vi "Get Configuration in File.vi"(8 "error in":errorcluster, 11 "Configuration File Path":path) -> (0 "error out":errorcluster, 3 "Configuration from File":T1={"Delay Mode"="On", "Trigger Position"=0.0, "Length Unit"="Percentage", "Record Length"=100.0} {"Record Length" format="%#_6g%"; "Trigger Position" format="%#_6ps"})   [LabVIEW 2025, in "Ni-Scope-Multirecords UI.lvlib"]
uses:
  Ni-Scope-Multirecords UI.lvlib
  <vilib>/JDP Science/JSONtext/String Subset.vi
  <vilib>/JDP Science/JSONtext/support/Strip Quotes and Unescape.vi
  <vilib>/JDP Science/JSONtext/support/Unescape JSON string.vi
  <vilib>/JDP Science/JSONtext/Parsing/Parse Full Path or Item Name.vi
  <vilib>/JDP Science/JSONtext/Offset/Find Item Locations by Path.vi
  <vilib>/ErrorRing/Error Ring.xnode
  <vilib>/JDP Science/JSONtext/JSONtext.lvlib
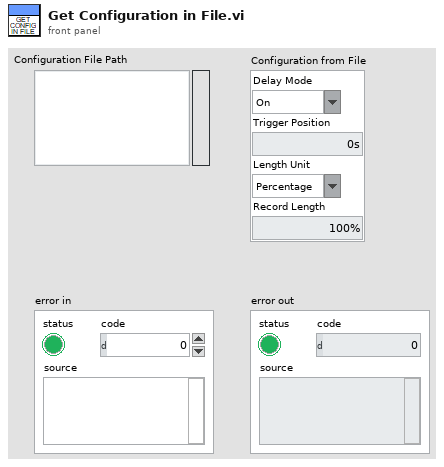
[diagram p1: front panel]
types:
  T1 = cluster{"Delay Mode":string, "Trigger Position":dbl, "Length Unit":string, "Record Length":dbl}
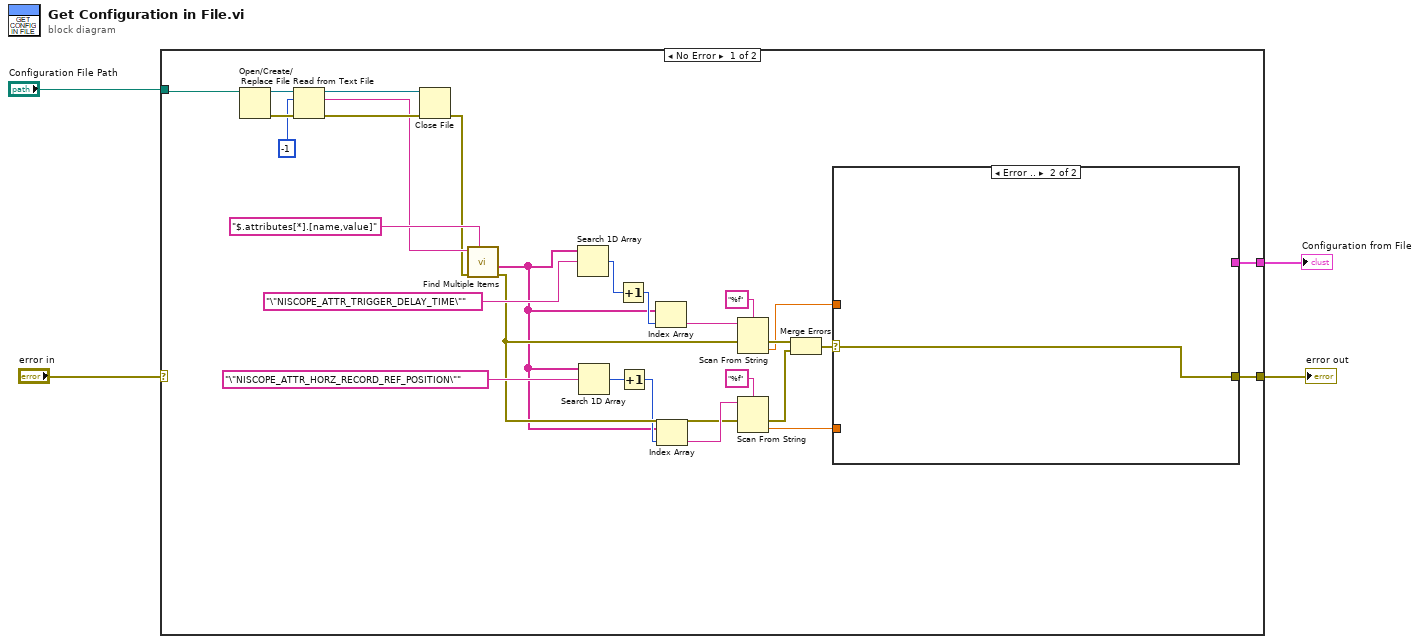
[diagram p0: block diagram]
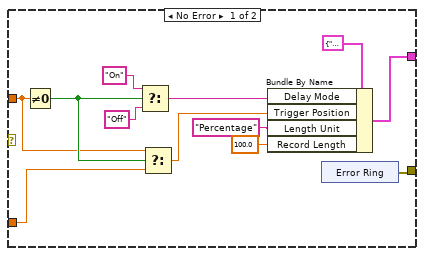
[diagram p2: hidden frame]
diagram:
  n1 = case shown="No Error" "error in" {
    selector: "error in" -> [_ w47]
    tunnel: [w9 w47] -> w3
    tunnel: "Configuration File Path" -> [w32 _]
    tunnel: [w10 _] -> w1
    frame No Error {
      n2 = Open/Create/Replace File(file path (use dialog)=w32) -> (refnum out=w30:refnum<file>, error out=w31:errorcluster)  [unwired: 5 in, 1 out]
      n3 = Read from Text File(file (use dialog)=w30, count=-1, error in=w31) -> (refnum out=w28:refnum<file>, text=w25:string, error out=w29:errorcluster)  [unwired: 1 in, 1 out]
      n4 = Close File(refnum=w28, error in=w29) -> (error out=w17:errorcluster)  [unwired: 1 out]
      n5 = call <vilib>:"Find Multiple Items.vi"("$Path or Item Name"="$.attributes[*].[name,value]", "error in (no error)"=w17, "JSON"=w25) -> ("error out"=w16:errorcluster, "<JSON>"=w5:string[])  [unwired: 5 in, 2 out]
      n6 = Search 1D Array(1D array=w5, element="\"NISCOPE_ATTR_TRIGGER_DELAY_TIME\"") -> (index of element=w7:i32)  [unwired: 1 in]
      n7 = Search 1D Array(1D array=w5, element="\"NISCOPE_ATTR_HORZ_RECORD_REF_POSITION\"") -> (index of element=w23:i32)  [unwired: 1 in]
      n8 = Increment(x=w7) -> (x+1=w8:i32)
      n9 = Increment(x=w23) -> (x+1=w6:i32)
      n10 = Index Array(array=w5, index=w8) -> (element=w21:string)
      n11 = Index Array(array=w5, index=w6) -> (element=w18:string)
      n12 = Scan From String(format string="%f", input string=w21, error in=w16) -> (error out=w15:errorcluster, output 1=w12:dbl)  [unwired: 2 in, 2 out]
      n13 = Scan From String(format string="%f", input string=w18, error in=w16) -> (error out=w14:errorcluster, output 1=w11:dbl)  [unwired: 2 in, 2 out]
      n14 = Merge Errors(w15, w14) -> (w13:errorcluster)
      n15 = case shown="Error .." w13 {
        selector: w13 -> [_ w46]
        tunnel: w12 -> [w38 _]
        tunnel: w11 -> [w37 _]
        tunnel: [w43 _] -> w10
        tunnel: [w33 w46] -> w9
        frame No Error {
          n16 = Not Equal To 0?(x=w38) -> (x != 0?=w39:bool)
          n17 = Select(t="On", s=w39, f="Off") -> (s? t:f=w40:string)
          n18 = Select(t=w38, s=w39, f=w37) -> (s? t:f=w36:dbl)
          n19 = Bundle By Name(cluster=T1 {"Delay Mode"="On", "Trigger Position"=0.0, "Length Unit"="Percentage", "Record Length"=100.0} ("Configuration from File"), "Delay Mode"=w40, "Trigger Position"=w36, "Length Unit"="Percentage", "Record Length"=100.0) -> (w43:T1)
          n20 = xnode "Error Ring"() -> ("error out"=w33:errorcluster)
        }
        frame Error {
        }
      }
    }
    frame Error {
    }
  }
  "error out" <- w3
  "Configuration from File" <- w1
